vi "Get Version.vi"(8 "error in (no error)":errorcluster) -> (0 "error out":errorcluster, 3 "version":string)   [LabVIEW 2020]
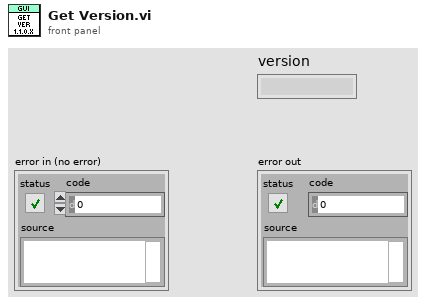
[diagram p1: front panel]
types:
  T1 = enum32{"invalid app kind", "Development System", "Run Time System", "Student Edition", "Embedded LabVIEW", "Evaluation", "Custom"}
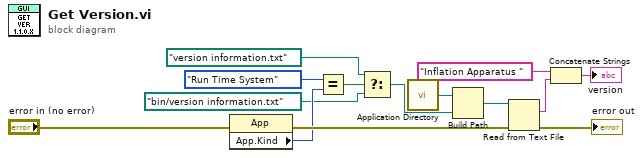
[diagram p0: block diagram]
diagram:
  n1 = property class="App"(error in="error in (no error)") -> (error out=w9:errorcluster, "App.Kind"=w8:T1)  [unwired: 1 in, 1 out]
  n2 = Equal?(x=T1."Run Time System" ("y"), y=w8) -> (x = y?=w11:bool)
  n3 = Select(t=path "version information.txt", s=w11, f=path "bin/version information.txt" ("name or relative path")) -> (s? t:f=w4:path)
  n4 = call <vilib>:"Application Directory.vi"() -> ("Application Directory"=w14:path)
  n5 = Build Path(base path=w14, name or relative path=w4) -> (appended path=w12:path)
  n6 = Read from Text File(file (use dialog)=w12, error in=w9) -> (text=w3:string, error out=→"error out":errorcluster)  [unwired: 2 in, 2 out]
  n7 = Concatenate Strings("Inflation Apparatus " ("string"), w3) -> (→"version":string)
